vi "PCA9586-Servo_Api.vi"(8 "Error In":errorcluster, 9 "角度":dbl, 10 "I2C Ref In":T1={"myRIO Reference"={"myRIO Model"=enum."Unknown", "myRIO Hardware Reference"={"Generic FPGA Reference"=refnum, "Allow multiple opens"=FALSE}}, "I2C Channels Enum"=enum."Not Connected", "I2C Configuration"={"I2C Transfer Rate"=enum."Fast mode (400 kbps)"}}, 11 "PWM腳位":T9(ring)) -> (0 "Error Out":errorcluster)   [LabVIEW 2019]
uses:
  <vilib>/myRIO/Instrument Drivers/Onboard IO/I2C/typedefs/I2C Reference.ctl
  <vilib>/myRIO/Common/Instrument Driver Framework/Utilities/typedefs/myRIO Generic Hardware Reference.ctl
  <vilib>/myRIO/Common/Instrument Driver Framework/Utilities/typedefs/Hardware Version Enum.ctl
  <vilib>/myRIO/Common/Instrument Driver Framework/Utilities/typedefs/myRIO v1.0 Reference.ctl
  <vilib>/myRIO/Common/Instrument Driver Framework/Utilities/typedefs/Generic FPGA Reference.ctl
  <vilib>/myRIO/Common/Instrument Driver Framework/myRIO v1.0/I2C/typedefs/I2C Channels Enum.ctl
  <vilib>/myRIO/Instrument Drivers/Onboard IO/I2C/typedefs/I2C Configuration.ctl
  <vilib>/myRIO/Instrument Drivers/Onboard IO/I2C/typedefs/I2C Transfer Rate.ctl
  <vilib>/myRIO/Instrument Drivers/Onboard IO/I2C/I2C.lvlib
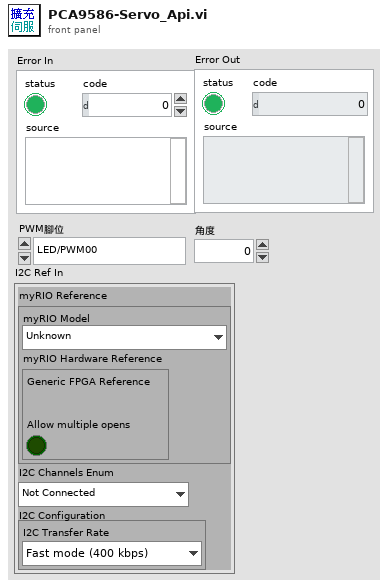
[diagram p1: front panel]
types:
  T1 = typedef "I2C.lvlib/I2C Reference.ctl" = cluster{"myRIO Reference":T2, "I2C Channels Enum":T6, "I2C Configuration":T7}
  T2 = typedef "myRIO Generic Hardware Reference.ctl" = cluster{"myRIO Model":T3, "myRIO Hardware Reference":T4}
  T3 = typedef "Hardware Version Enum.ctl" = enum16{"Unknown", "myRIO-1900", "myRIO-1950", "roboRIO", "NI ELVIS RIO CM", "ELVIS III"}
  T4 = typedef "myRIO v1.0 Reference.ctl" = cluster{"Generic FPGA Reference":T5, "Allow multiple opens":bool}
  T5 = typedef "Generic FPGA Reference.ctl" = refnum<k20>
  T6 = typedef "I2C Channels Enum.ctl" = enum16{"Not Connected", "A/I2C", "B/I2C", "I2C/I2C"}
  T7 = typedef "I2C.lvlib/I2C Configuration.ctl" = cluster{"I2C Transfer Rate":T8}
  T8 = typedef "I2C.lvlib/I2C Transfer Rate.ctl" = enum16{"Standard mode (100 kbps)", "Fast mode (400 kbps)"}
  T9 = enum16{"LED/PWM00", "LED/PWM01", "LED/PWM02", "LED/PWM03", "LED/PWM04", "LED/PWM05", "LED/PWM06", "LED/PWM07", "LED/PWM08", "LED/PWM09", "LED/PWM10", "LED/PWM11", "LED/PWM12", "LED/PWM13", "LED/PWM14", "LED/PWM15"}
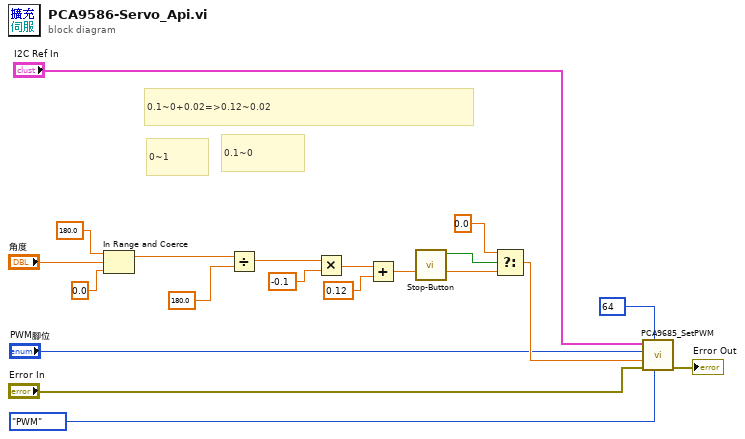
[diagram p0: block diagram]
diagram:
  # "0.1~0+0.02=>0.12~0.02"
  # "0.1~0"
  # "0~1"
  n1 = In Range and Coerce(upper limit=180.0, x="角度", lower limit=0.0) -> (coerced(x)=w16:dbl)  [unwired: 1 out]
  n2 = Divide(x=w16, y=180.0) -> (x/y=w14:dbl)
  n3 = Multiply(x=w14, y=-0.1) -> (x*y=w12:dbl)
  n4 = Add(x=w12, y=0.12) -> (x+y=w10:dbl)
  n5 = call "Stop-Button.vi"() -> ("顯示按下?"=w8:bool)  [unwired: 10 in, 1 out]
  n6 = Select(t=0.0, s=w8, f=w10) -> (s? t:f=w7:dbl)
  n7 = call "PCA9685_SetPWM.vi"("控制模式"=enum16{"PWM", "LED ON", "LED OFF"}."PWM", "驅動板位址(0x40)"=u8 64, "Error In"="Error In", "Duty Cycle(0~1)"=w7, "PWM腳位"="PWM腳位", "I2C Ref In"="I2C Ref In") -> ("Error Out"=→"Error Out":errorcluster)  [unwired: 4 in, 1 out]
